vi "Get Oldest File.vi"(8 "Error In":errorcluster, 10 "File Names":string[](array[string]), 11 "Folder":path) -> (0 "Error Out":errorcluster, 3 "Oldest File":path)   [LabVIEW 2015, in "Logger.lvlib" / "File.lvlib"]
uses:
  File.lvlib
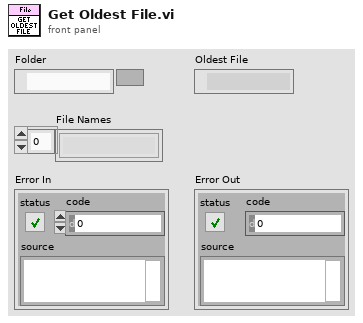
[diagram p1: front panel]
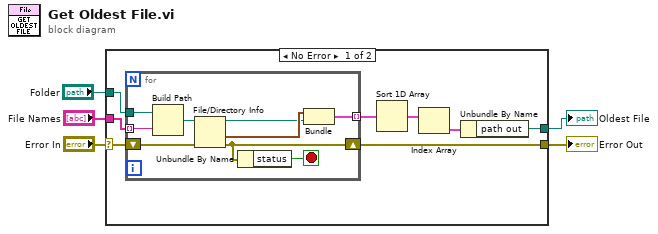
[diagram p0: block diagram]
diagram:
  n1 = case shown="No Error" "Error In" {
    selector: "Error In" -> [w6 w23]
    tunnel: "Folder" -> [w10 w24]
    tunnel: "File Names" -> [w9 _]
    tunnel: [w8 w24] -> w3
    tunnel: [w7 w23] -> w2
    frame No Error {
      n2 = for {
        tunnel: w9 -> [w21] mode=indexing
        tunnel: w10 -> [w20]
        tunnel: [w16] -> w13 mode=indexing
        shift-right: [w15] -> w7
        shift-left: w6 -> [w22]
        stop <- w14 stop-if-true
        n3 = Build Path(base path=w20, name or relative path=w21) -> (appended path=w19:path)
        n4 = File/Directory Info(path=w19, error in=w22) -> (path out=w17:path, last mod=w18:timestamp, error out=w15:errorcluster)  [unwired: 4 out]
        n5 = Unbundle By Name(w15) -> ("status"=w14:bool)
        n6 = Bundle("last mod"=w18, "path out"=w17) -> (w16:cluster{"last mod":timestamp, "path out":path})  [unwired: 1 in]
      }
      n7 = Sort 1D Array(array=w13) -> (sorted array=w12:cluster{"last mod":timestamp, "path out":path}[])
      n8 = Index Array(array=w12) -> (element=w11:cluster{"last mod":timestamp, "path out":path})  [unwired: 1 in]
      n9 = Unbundle By Name(w11) -> ("path out"=w8:path)
    }
    frame Error {
    }
  }
  "Oldest File" <- w3
  "Error Out" <- w2
